vi "DB test.vi"() -> ()   [LabVIEW 2020]
panel:
  in  "DB path":path
  out "DB Data":T1
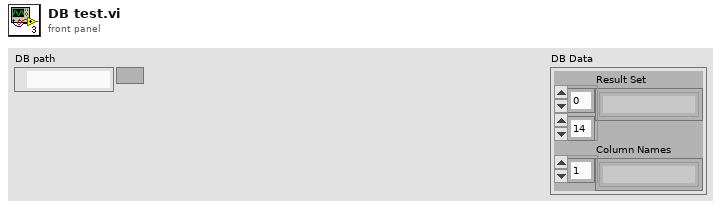
[diagram p1: front panel]
types:
  T1 = cluster{"Result Set":string[][], "Column Names":string[]}
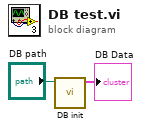
[diagram p0: block diagram]
diagram:
  n1 = call "DB init.vi"("DB path"="DB path") -> ("DB Data"=→"DB Data":T1)  [unwired: 9 in, 1 out]
